vi "QueryMirror.vi"(8 "error in (no error)":errorcluster, 10 "Mirror":enum16{"Entrance Mirror", "Exit Mirror"}(ring), 11 "Spectrometer in":refnum<class "Spectrometer.lvclass">) -> (0 "error out":errorcluster, 3 "Spectrometer out":refnum<class "Spectrometer.lvclass">)   [LabVIEW 2023, in "Spectrometer.lvclass"]
uses:
  Spectrometer.lvclass
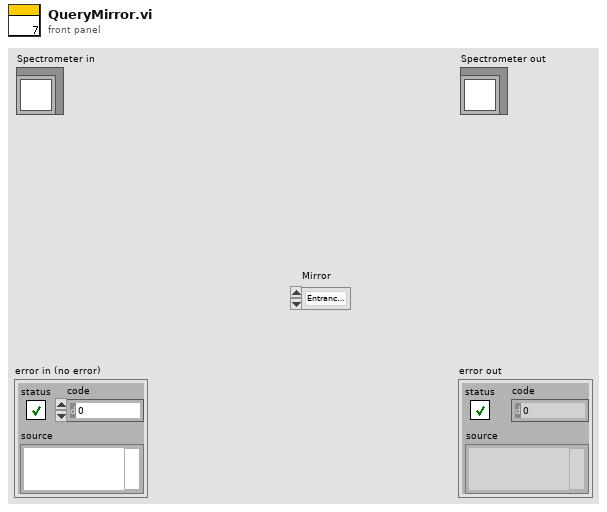
[diagram p1: front panel]
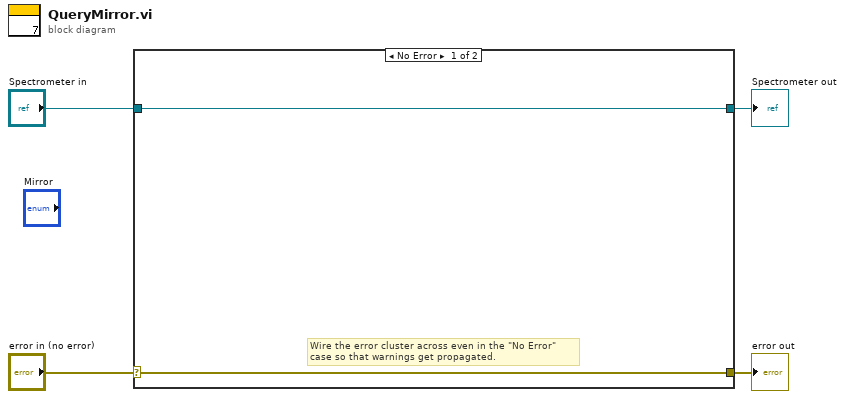
[diagram p0: block diagram]
diagram:
  n1 = case shown="No Error" "error in (no error)" {
    selector: "error in (no error)" -> [w5 w8]
    tunnel: [w5 w8] -> w3
    tunnel: [w6 w7] -> w1
    tunnel: "Spectrometer in" -> [w6 w7]
    frame No Error {
      # "Wire the error cluster across even in the \"No Error\"\ncase so that warnings get propagated."
    }
    frame Error {
    }
  }
  "error out" <- w3
  "Spectrometer out" <- w1
